vi "Variant to Class.vi"(8 "error in (no error)":errorcluster, 10 "Data in":variant, 11 "VIPC Apply Node in":refnum<class "VIPC Apply Node.lvclass">) -> (0 "error out":errorcluster, 2 "Data Out":variant, 3 "VIPC Apply Node out":refnum<class "VIPC Apply Node.lvclass">)   [LabVIEW 2014, in "VIPC Apply Node.lvclass"]
uses:
  VIPC Apply Node.lvclass
  Shared/Controls/VIPC Apply - STYP.ctl
  VIPC Apply Node.lvclass/VIPC Apply Node.ctl
  Classes/Build Job/Build Job.lvclass
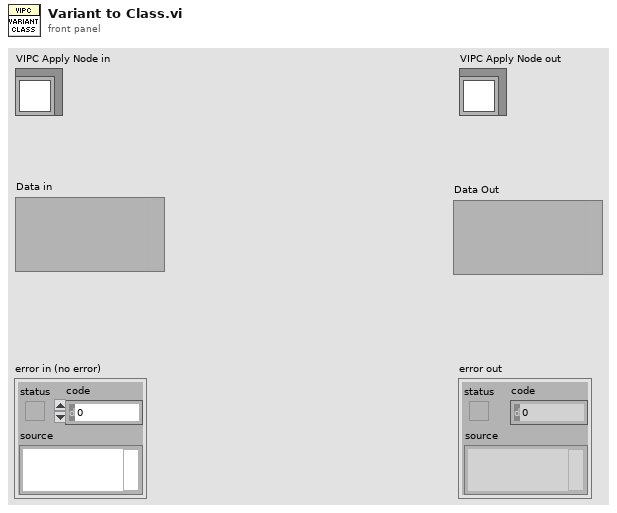
[diagram p1: front panel]
types:
  T1 = typedef "VIPC Apply - STYP.ctl" = cluster{"VIPC Path":string, "LabVIEW Version":string}
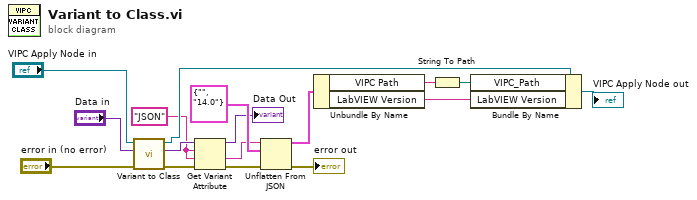
[diagram p0: block diagram]
diagram:
  w5 = "JSON" ("name")
  n1 = call-parent "Variant to Class.vi"("error in (no error)"="error in (no error)", "Data in"="Data in", "Build Job in"="VIPC Apply Node in") -> ("error out"=w4:errorcluster, "Data Out"=w7:variant, "Build Job out"=w8:refnum<class "VIPC Apply Node.lvclass">)  [unwired: 6 in]
  n2 = Get Variant Attribute(Variant=w7, name=w5, default value (empty Variant)=w5, error in=w4) -> (duplicate Variant=→"Data Out":variant, value=w10:string, error out=w9:errorcluster)  [unwired: 1 out]
  n3 = Unflatten From JSON(JSON string=w10, type and defaults=T1 {"VIPC Path"="", "LabVIEW Version"="14.0"} ("VIPC Apply"), error in (no error)=w9) -> (value=w12:T1, error out=→"error out":errorcluster)  [unwired: 4 in]
  n4 = Unbundle By Name(w12) -> ("VIPC Path"=w13:string, "LabVIEW Version"=w1:string)
  n5 = String To Path(string=w13) -> (path=w14:path)
  n6 = Bundle By Name(cluster=w8, "VIPC_Path"=w14, "LabVIEW Version"=w1) -> (→"VIPC Apply Node out":refnum<class "VIPC Apply Node.lvclass">)
